vi "Pre Launch Init.vi"(11 "Syringe in":refnum<class "Syringe Line.lvclass">) -> (0 "error out":errorcluster, 3 "Syringe out":refnum<class "Syringe Line.lvclass">)   [LabVIEW 2015, in "cRIO-Carbondioxide.lvlib" / "CO2-Actor.lvlib" / "Syringe Line.lvclass"]
doc: "(<B>Filename</B>: Actor Framework.lvlib:Actor.lvclass:Pre Launch Init.vi)\n\nDefines behavior that occurs after the Launch Actor method is invoked but before the actor's Actor Core method begins running.\n\nThe Pre Launch Init method is guaranteed to finish before the Launch Actor method returns to its caller and before the actor itself receives any messages. Any references that the Pre Launch Init method obtains are guaranteed to have the same lifetime as the actor itself. Any errors that the Pre Launch Init method returns will abort the launch.\n\nBy default, this method does nothing. A descendant class may override it to define behavior."
uses:
  Syringe Line.lvclass
  Syringe Line.lvclass/Syringe Line.ctl
  <vilib>/ActorFramework/Actor/Actor.lvclass/Actor.ctl
  <vilib>/ActorFramework/Message Enqueuer/Message Enqueuer.lvclass/Message Enqueuer.ctl
  <vilib>/ActorFramework/Message Enqueuer/Enqueue.vi
  <vilib>/ActorFramework/Actor/Read Self Enqueuer.vi
  <vilib>/ActorFramework/Message Enqueuer/Init from Existing Queue.vi
  <vilib>/ActorFramework/Message Priority Queue/Priority Enqueue.vi
  CO2 Actor/CO2 Actor.lvclass
  Syringe Line Messages/Set Valve Capillary Line Enqueuer Msg/Set Valve Capillary Line Enqueuer Msg.lvclass
  CO2 Actor Messages/Launch Nested Actors Msg/Launch Nested Actors Msg.lvclass
  <vilib>/ActorFramework/Message Enqueuer/Message Enqueuer.lvclass
  <vilib>/ActorFramework/Actor/Actor.lvclass
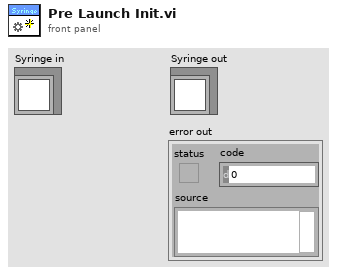
[diagram p1: front panel]
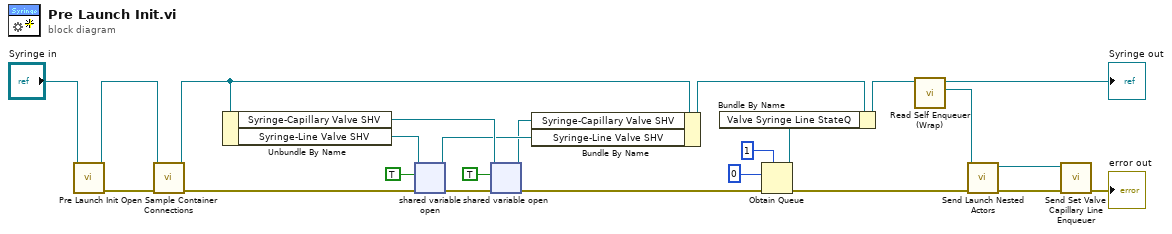
[diagram p0: block diagram]
diagram:
  n1 = call-parent "Pre Launch Init.vi"("CO2 Actor in"="Syringe in") -> ("error out"=w23:errorcluster, "CO2 Actor out"=w22:refnum<class "Syringe Line.lvclass">)  [unwired: 9 in]
  n2 = call "Open Sample Container Connections.vi"("error in (no error)"=w23, "Syringe in"=w22) -> ("error out"=w18:errorcluster, "Syringe out"=w19:refnum<class "Syringe Line.lvclass">)  [unwired: 8 in]
  n3 = Unbundle By Name(w19) -> ("Syringe-Capillary Valve SHV"=w16:refnum<k21>, "Syringe-Line Valve SHV"=w13:refnum<k21>)
  n4 = shared-variable-open(w13, w18, TRUE) -> (w12:refnum<k21>, w17:errorcluster)  [unwired: 1 in]
  n5 = shared-variable-open(w16, w17, TRUE) -> (w11:refnum<k21>, w5:errorcluster)  [unwired: 1 in]
  n6 = Bundle By Name(cluster=w19, "Syringe-Capillary Valve SHV"=w11, "Syringe-Line Valve SHV"=w12) -> (w10:refnum<class "Syringe Line.lvclass">)
  n7 = Obtain Queue(max queue size (-1, unlimited)=1, element data type=u16 0, error in (no error)=w5) -> (queue out=w3:refnum<queue>, error out=w4:errorcluster)  [unwired: 2 in, 1 out]
  n8 = Bundle By Name(cluster=w10, "Valve Syringe Line StateQ"=w3) -> (w6:refnum<class "Syringe Line.lvclass">)
  n9 = call "Read Self Enqueuer (Wrap).vi"("CO2 Actor in"=w6) -> ("Actor Framework:Message Enqueuer"=w20:refnum<class "Message Enqueuer.lvclass">, "CO2 Actor out"=→"Syringe out":refnum<class "Syringe Line.lvclass">)  [unwired: 9 in]
  n10 = call "Send Launch Nested Actors.vi"("error in (no error)"=w4, "Message Enqueuer"=w20) -> ("error out"=w9:errorcluster, "Message Enqueuer out"=w7:refnum<class "Message Enqueuer.lvclass">)  [unwired: 8 in]
  n11 = call "Send Set Valve Capillary Line Enqueuer.vi"("error in (no error)"=w9, "Message Enqueuer"=w7) -> ("error out"=→"error out":errorcluster)  [unwired: 8 in, 1 out]
